vi "_PC_Pub_DBL2Boolean.vi"(1 "DBL":dbl=3.14 format="%.2f") -> (0 "Boolean array":bool[](array[boolean]))   [LabVIEW 2018]
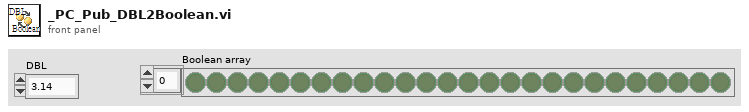
[diagram p1: front panel]
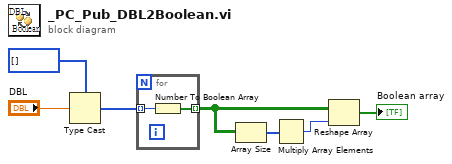
[diagram p0: block diagram]
diagram:
  n1 = Type Cast(type=u32[] [], x="DBL") -> (*(type *) &x=w2:u32[])
  n2 = for {
    tunnel: w2 -> [w9] mode=indexing
    tunnel: [w8] -> w5 mode=indexing
    n3 = Number To Boolean Array(number=w9) -> (Boolean array=w8:bool[])
  }
  n4 = Array Size(array=w5) -> (size(s)=w6:i32[])
  n5 = Multiply Array Elements(1:w6) -> (0:w4:i32)
  n6 = Reshape Array(w5, w4) -> (→"Boolean array":bool[])
